vi "GetStateMask.vi"(8 "error in (no error)":errorcluster caption="Fehler (Eingang, kein Fehler)", 11 "device":u32) -> (0 "error out":errorcluster caption="Fehler (Ausgang)", 2 "function return":u32(ring), 3 "mask":u16)   [LabVIEW 2015, in "IRB.lvlib"]
doc: "irb_result IRB_EXPORT irb_get_state_mask(irb_device* device, uint16_t* mask);"
uses:
  IRB.lvlib
  IRB.dll
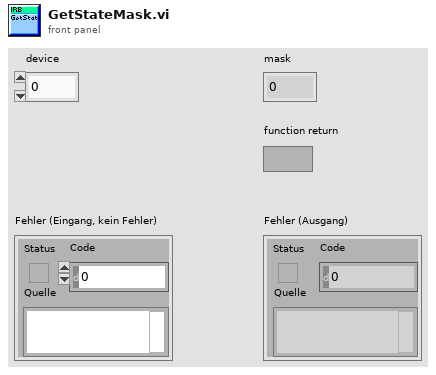
[diagram p1: front panel]
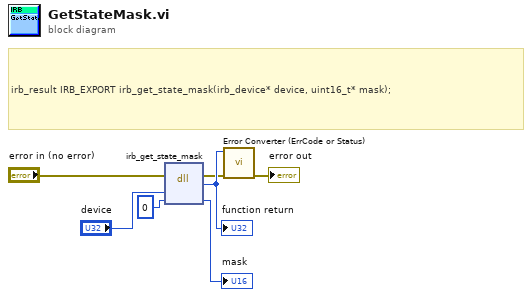
[diagram p0: block diagram]
diagram:
  # "irb_result IRB_EXPORT irb_get_state_mask(irb_device* device, uint16_t* mask);"
  n1 = dll-call lib="C:/LabView/IRB/x86_32/IRB.*" fn="irb_get_state_mask"(error in="error in (no error)", "device"="device", "mask"=u16 0) -> (error out=w2:errorcluster, "return type"=w7:u32, "mask"=→"mask":u16)  [unwired: 3 in, 1 out]
  "function return" <- w7
  n2 = call "Error Converter (ErrCode or Status).vi"("error in (no error)"=w2, "error code"=w7) -> ("error out"=→"error out":errorcluster)  [unwired: 9 in]
